vi "OAT Tachless Update Cursor After Refine.vi"(7 "refined profile":T1 {"speed [RPM]" format="%.2f"; "time [s]" format="%.2f"}, 10 "Chkpnt Order":dbl format="%.2f", 11 "cursors":T2(array[cluster]) {"Location"."Y" format="%.2f"; "Location"."X" format="%.2f"}) -> (3 "cursors out":T2(array[cluster]) {"Location"."Y" format="%.2f"; "Location"."X" format="%.2f"})   [LabVIEW 2017, in "SoundVib_Tachless.lvlib"]
uses:
  <vilib>/addons/Sound and Vibration/Order Analysis/Tachless/SoundVib_Tachless.lvlib
  <vilib>/addons/Sound and Vibration/Order Analysis/Tach Process/SubVIs/speed profile.ctl
  <vilib>/addons/Sound and Vibration/Order Analysis/Tach Process/SoundVib_TachProcess.lvlib
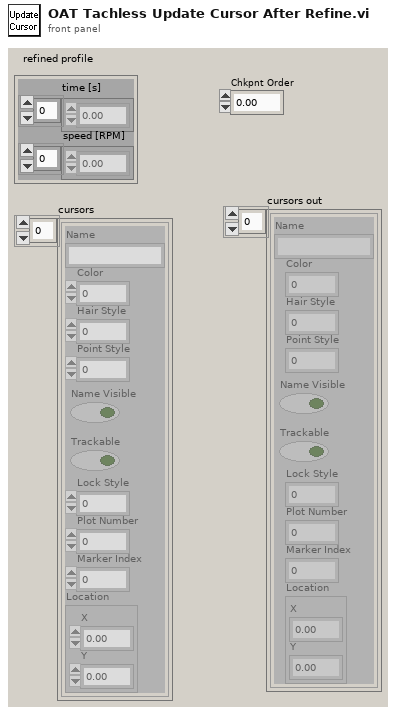
[diagram p1: front panel]
types:
  T1 = typedef "SoundVib_TachProcess.lvlib/speed profile.ctl" = cluster{"time [s]":dbl[], "speed [RPM]":dbl[]}
  T2 = cluster{"Name":string, "Color":u32, "Hair Style":u8, "Point Style":u8, "Name Visible":bool, "Trackable":bool, "Lock Style":u32, "Plot Number":u32, "Marker Index":i32, "Location":cluster{"X":dbl, "Y":dbl}}[]
  T3 = cluster{"Name":string, "Color":u32, "Hair Style":u8, "Point Style":u8, "Name Visible":bool, "Trackable":bool, "Lock Style":u32, "Plot Number":u32, "Marker Index":i32, "Location":cluster{"X":dbl, "Y":dbl}}
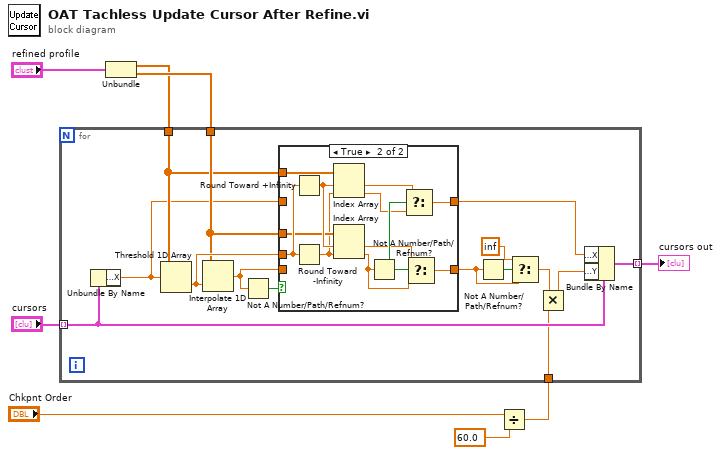
[diagram p0: block diagram]
diagram:
  n1 = Unbundle("refined profile") -> ("time [s]"=w5:dbl[], "speed [RPM]"=w6:dbl[])
  n2 = Divide(x="Chkpnt Order", y=60.0) -> (x/y=w2:dbl)
  n3 = for {
    tunnel: "cursors" -> [w23] mode=indexing
    tunnel: w5 -> [w16]
    tunnel: w6 -> [w17]
    tunnel: [w22] -> w8 mode=indexing
    tunnel: w2 -> [w10]
    n4 = Unbundle By Name(w23) -> ("Location.X"=w15:dbl)
    n5 = Threshold 1D Array(2:w15, 3:w16) -> (0:w18:dbl)  [unwired: 1 in]
    n6 = Interpolate 1D Array(1:w18, 2:w17) -> (0:w14:dbl)
    n7 = Not A Number/Path/Refnum?(number/path/refnum=w14) -> (NaN/Path/Refnum?=w19:bool)
    n8 = case shown="True" w19 {
      tunnel: w18 -> [_ w36]
      tunnel: w17 -> [_ w28]
      tunnel: [w24 w34] -> w13
      tunnel: w16 -> [_ w30]
      tunnel: [w25 w31] -> w12
      tunnel: w15 -> [w25 _]
      tunnel: w14 -> [w24 _]
      frame False {
      }
      frame True {
        n9 = Round Toward +Infinity(x=w36) -> (ceil(x): smallest int >= x=w37:dbl)
        n10 = Round Toward -Infinity(1:w36) -> (0:w27:dbl)
        n11 = Index Array(array=w30, index #1=w37, index #2=w27) -> (element #1=w32:dbl, element #2=w29:dbl)
        n12 = Index Array(array=w28, index #1=w37, index #2=w27) -> (element #1=w33:dbl, element #2=w26:dbl)
        n13 = Not A Number/Path/Refnum?(number/path/refnum=w26) -> (NaN/Path/Refnum?=w35:bool)
        n14 = Select(t=w32, s=w35, f=w29) -> (s? t:f=w31:dbl)
        n15 = Select(t=w33, s=w35, f=w26) -> (s? t:f=w34:dbl)
      }
    }
    n16 = Not A Number/Path/Refnum?(number/path/refnum=w13) -> (NaN/Path/Refnum?=w21:bool)
    n17 = Select(t=inf, s=w21, f=w13) -> (s? t:f=w9:dbl)
    n18 = Multiply(x=w9, y=w10) -> (x*y=w11:dbl)
    n19 = Bundle By Name(cluster=w23, "Location.X"=w12, "Location.Y"=w11) -> (w22:T3)
  }
  "cursors out" <- w8
